vi "AS01.vi"() -> ()   [LabVIEW 2017]
panel:
  in  "x>=y2":dbl
  in  "x<=y2":dbl
  out "Boolean 2":bool
  out "Celcius":dbl
  out "C 3":dbl
  out "Celcius":dbl(slide) scale=-50.0..100.0
  in  "Fahrenheit":dbl(knob) scale=-58.0..212.0
  out "LED 2":bool
  in  "Numeric 2":dbl
  in  "Numeric":dbl
  out "Boolean":bool
  out "F":dbl
  out "C":dbl
  out "F":dbl(slide) scale=-50.0..100.0
  in  "C":dbl(knob) scale=-58.0..212.0
  out "LED 1":bool
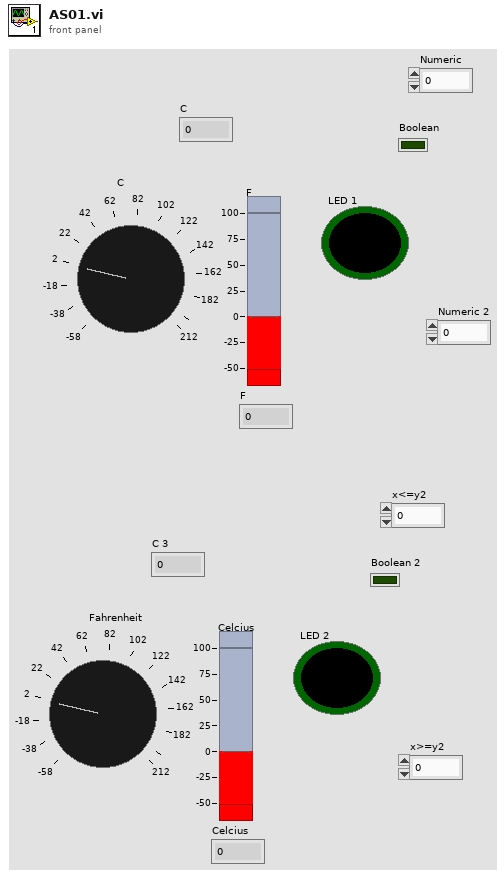
[diagram p1: front panel]
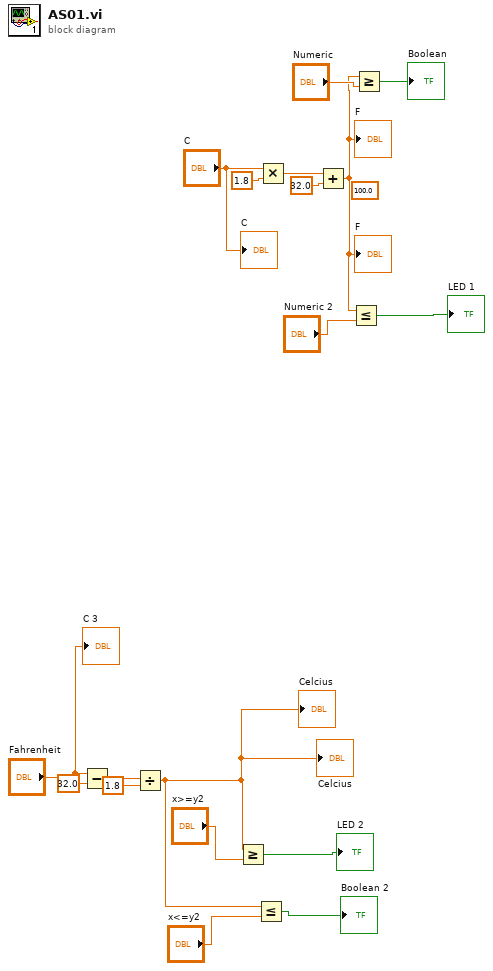
[diagram p0: block diagram]
diagram:
  (unwired) 100.0 ("y")
  n1 = Subtract(x="Fahrenheit", y=32.0) -> (x-y=w7:dbl)
  n2 = Divide(x=w7, y=1.8) -> (x/y=w3:dbl)
  "Celcius" <- w3
  "Celcius" <- w3
  n3 = Greater Or Equal?(x=w3, y="x>=y2") -> (x >= y?=→"LED 2":bool)
  n4 = Less Or Equal?(x=w3, y="x<=y2") -> (x <= y?=→"Boolean 2":bool)
  n5 = Multiply(x="C", y=1.8 ("x")) -> (x*y=w18:dbl)
  n6 = Add(x=w18, y=32.0) -> (x+y=w11:dbl)
  "F" <- w11
  "F" <- w11
  n7 = Less Or Equal?(x=w11, y="Numeric 2") -> (x <= y?=→"LED 1":bool)
  n8 = Greater Or Equal?(x=w11, y="Numeric") -> (x >= y?=→"Boolean":bool)
  "C" <- "C"
  "C 3" <- "Fahrenheit"
